vi "Get Bounds (Float).vi"(8 "error in (no error)":errorcluster, 10 "Feature":string, 11 "Camera in":refnum<class "Camera.lvclass">) -> (0 "error out":errorcluster, 1 "Max":dbl, 2 "Min":dbl, 3 "Camera":refnum<class "Camera.lvclass">)   [LabVIEW 2020, in "Camera.lvclass"]
uses:
  Camera.lvclass
  Camera.lvclass/Camera.ctl
  bin/gindustrialcam_32-1.dll
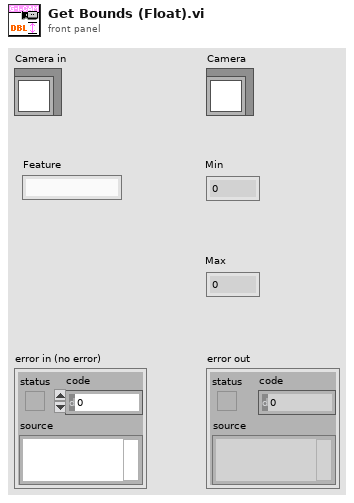
[diagram p1: front panel]
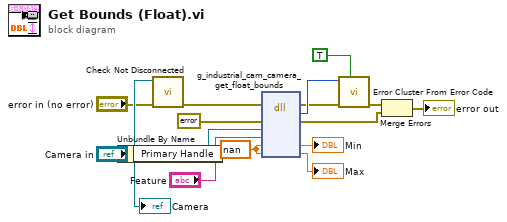
[diagram p0: block diagram]
diagram:
  w2 = nan ("Value In")
  n1 = Unbundle By Name("Camera in") -> ("Primary Handle"=w10:refnum<data-value>)
  n2 = call "Check Not Disconnected.vi"("error in (no error)"="error in (no error)", "Camera in"="Camera in") -> ("error out"=w11:errorcluster)  [unwired: 9 in]
  n3 = dll-call lib="C:/serenial/lib/g-industrial-camera/LabVIEW/g_industrial_cam/bin/gindustrialcam_*-1.*" fn="g_industrial_cam_camera_get_float_bounds"(error in=w11, "err"=errorcluster {"status"=FALSE, "code"=0, "source"=""} ("error constant"), "edvr"=w10, "feature"="Feature", "min"=w2, "max"=w2) -> (error out=w4:errorcluster, "Mg_Error"=w5:i32, "err"=w7:errorcluster, "min"=→"Min":dbl, "max"=→"Max":dbl)  [unwired: 4 in, 1 out]
  n4 = call <vilib>:"Error Cluster From Error Code.vi"("show call chain? (False)"=TRUE, "error in (no error)"=w4, "error code (0)"=w5) -> ("error out"=w6:errorcluster)  [unwired: 6 in]
  n5 = Merge Errors(w6, w7) -> (→"error out":errorcluster)
  "Camera" <- "Camera in"
